vi "Read Target.vi"(11 "ProjectItem in":refnum<class "ProjectItem.lvclass">) -> (2 "Target":string, 3 "ProjectItem out":refnum<class "ProjectItem.lvclass">)   [LabVIEW 2019, in "SolutionBuilder.lvlib" / "ProjectItem.lvclass"]
uses:
  ProjectItem.lvclass
  ProjectItem.lvclass/ProjectItem.ctl
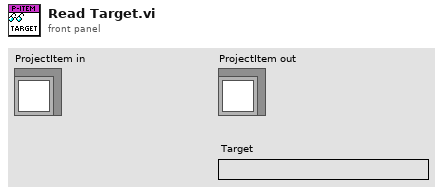
[diagram p1: front panel]
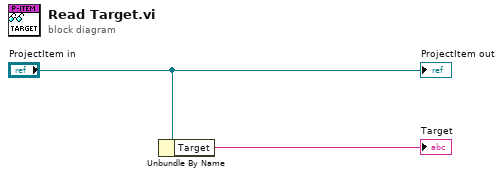
[diagram p0: block diagram]
diagram:
  n1 = Unbundle By Name("ProjectItem in") -> ("Target"=→"Target":string)
  "ProjectItem out" <- "ProjectItem in"
